vi "read text file.vi"() -> ()   [LabVIEW 2016]
panel:
  in  "File Path":path
  out "File Contents":string
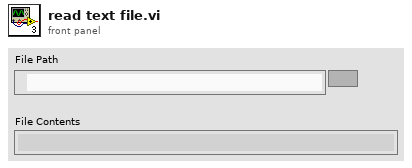
[diagram p1: front panel]
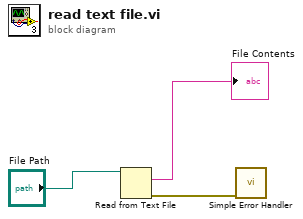
[diagram p0: block diagram]
diagram:
  n1 = Read from Text File(file (use dialog)="File Path") -> (text=→"File Contents":string, error out=w2:errorcluster)  [unwired: 3 in, 2 out]
  n2 = call <vilib>:"Simple Error Handler.vi"("error in (no error)"=w2) -> ()  [unwired: 4 in, 5 out]
